vi "SystemExec.vi"() -> ()   [LabVIEW 2019, in "ctet_other User.lvlib"]
uses:
  ctet_other User.lvlib
panel:
  out "standard error":string
  out "return code":i32
  out "standard output":string
  out "error out":errorcluster
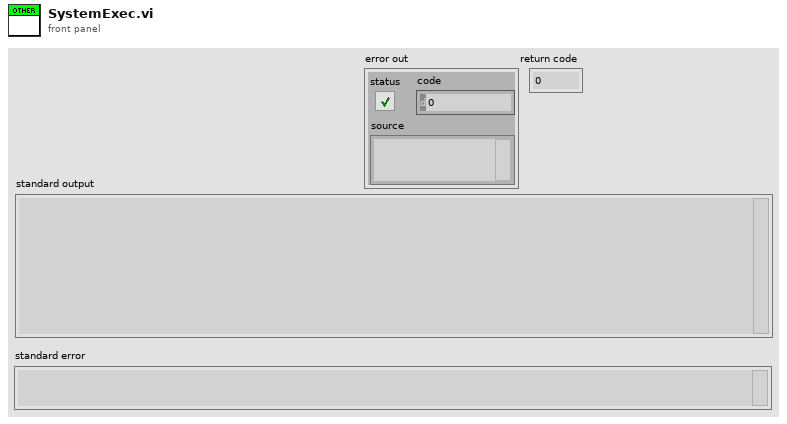
[diagram p1: front panel]
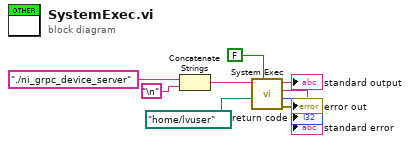
[diagram p0: block diagram]
diagram:
  n1 = Concatenate Strings("./ni_grpc_device_server" ("standard input"), "\n") -> (w1:string)
  n2 = call <vilib>:"System Exec.vi"("wait until completion? (T)"=FALSE, "working directory"=path "/home/lvuser", "command line"=w1) -> ("error out"=→"error out":errorcluster, "return code"=→"return code":i32, "standard error"=→"standard error":string, "standard output"=→"standard output":string)  [unwired: 5 in]
